vi "1_计算器V1.vi"() -> ()   [LabVIEW 2016]
uses:
  <vilib>/regexp/Match Regular Expression.xnode
panel:
  out "组合框":string(combo)
  in  "按键":T1
  out "Y":string
  out "X":string
  out "B":string
  out "A":string
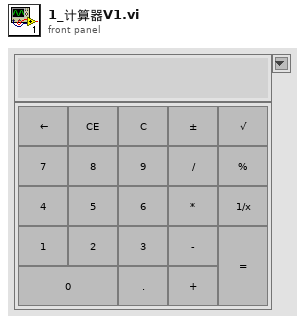
[diagram p1: front panel]
types:
  T1 = cluster{"7":bool, "8":bool, "9":bool, "4":bool, "5":bool, "6":bool, "1":bool, "2":bool, "3":bool, "0":bool, "/":bool, "*":bool, "-":bool, "+":bool, "=":bool, ".":bool, "±":bool, "CE":bool, "C":bool, "←":bool, "√":bool, "1/x":bool, "%":bool}
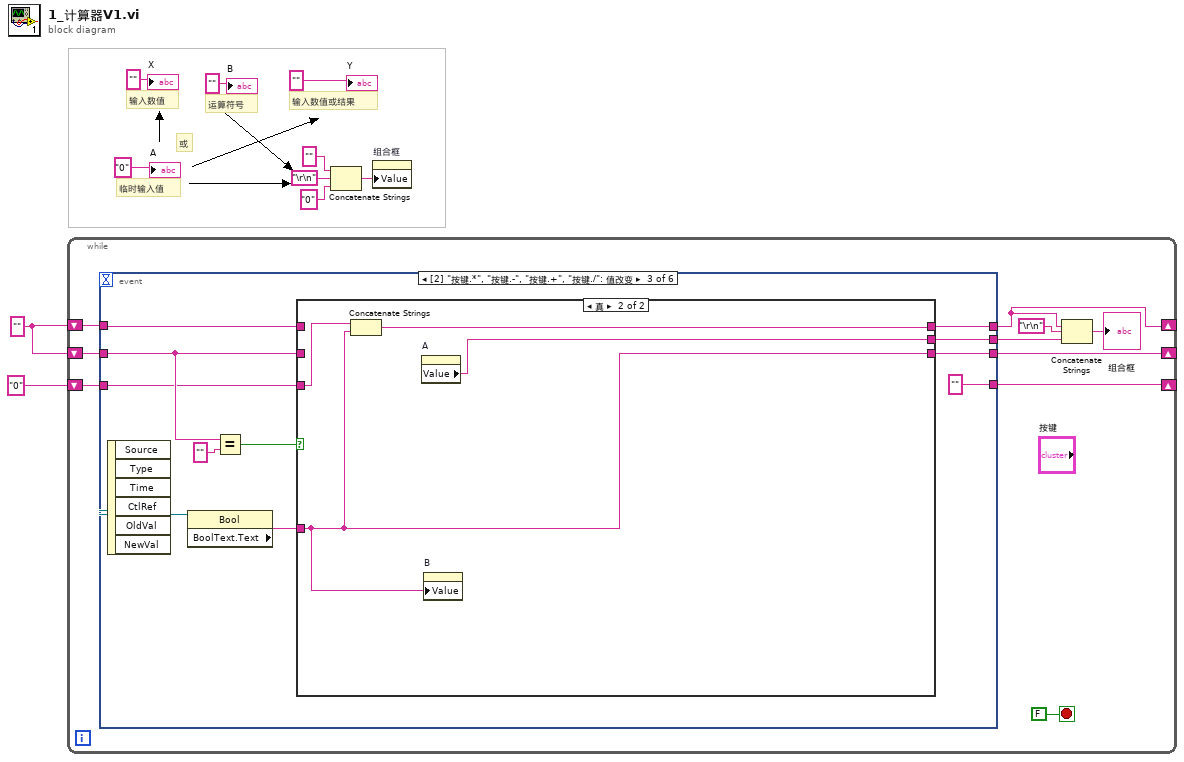
[diagram p0: block diagram]
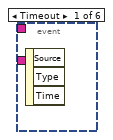
[diagram p2: hidden frame]
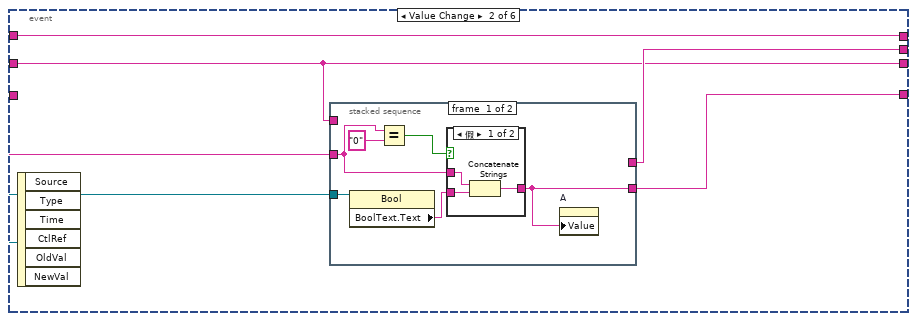
[diagram p3: hidden frame]
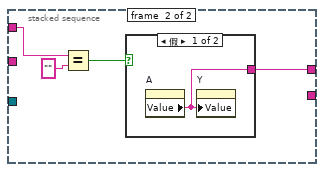
[diagram p5: hidden frame]
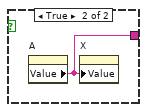
[diagram p6: hidden frame]
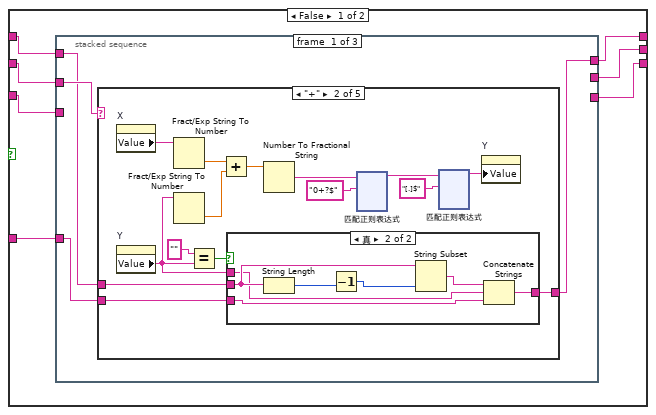
[diagram p7: hidden frame]
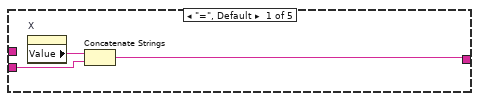
[diagram p8: hidden frame]
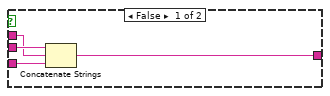
[diagram p9: hidden frame]
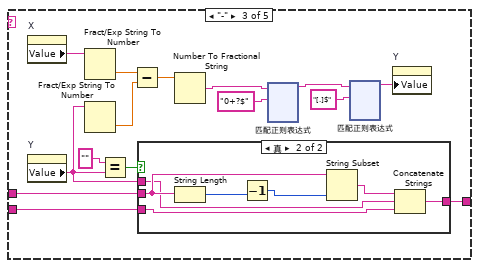
[diagram p10: hidden frame]
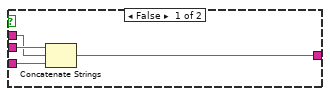
[diagram p11: hidden frame]
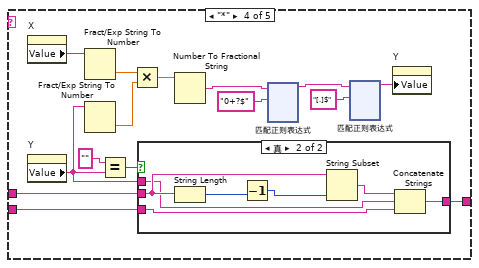
[diagram p12: hidden frame]
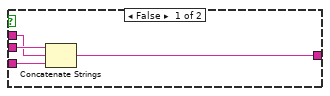
[diagram p13: hidden frame]
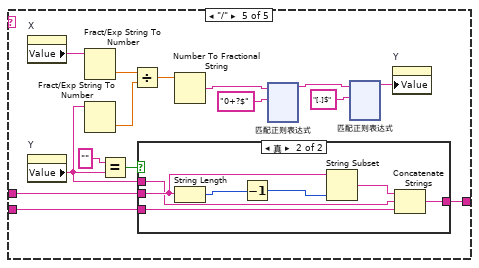
[diagram p14: hidden frame]
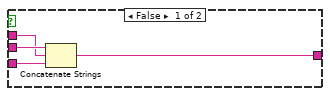
[diagram p15: hidden frame]
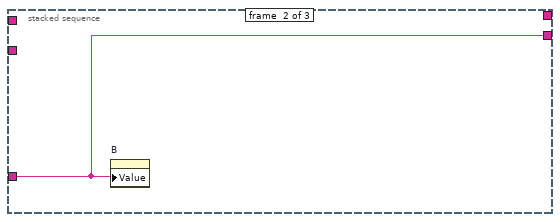
[diagram p16: hidden frame]
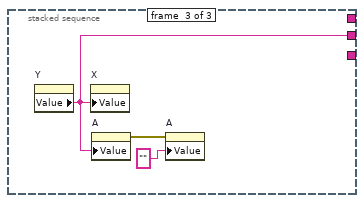
[diagram p17: hidden frame]
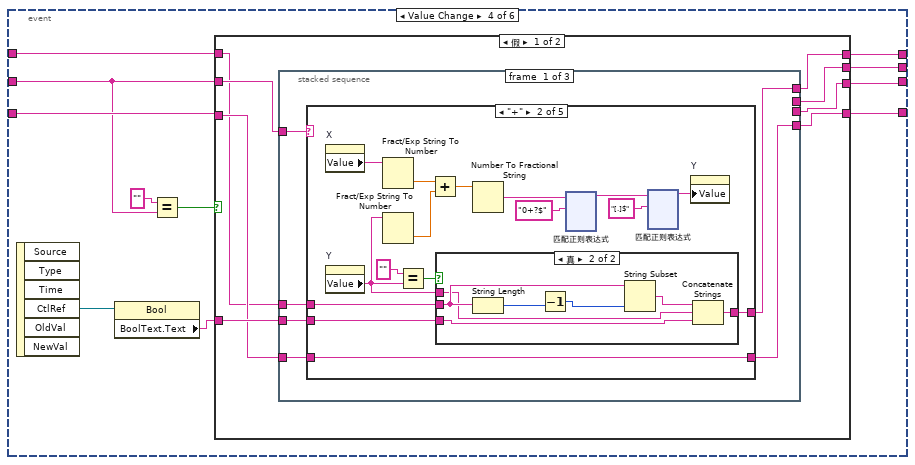
[diagram p18: hidden frame]
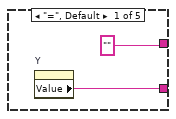
[diagram p19: hidden frame]
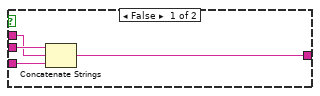
[diagram p20: hidden frame]
diagram:
  w1 = ""
  # "或"
  # "输入数值或结果"
  # "输入数值"
  # "运算符号"
  # "临时输入值"
  n1 = while {
    shift-right: [w18] -> _
    shift-left: "0" -> [w19]
    shift-right: [w16] -> _
    shift-left: w1 -> [w17]
    shift-right: [w12] -> _
    shift-left: w1 -> [w15]
    stop <- FALSE stop-if-true
    n2 = event shown="[2] \"按键.*\", \"按键.-\", \"按键.+\", \"按键./\": 值改变" {
      selector: _ -> [_ _ _ _ _ _]
      dyn-events: _ -> [_ _ _ _ _ _]
      timeout: _ -> [_ _ _ _ _ _]
      tunnel: w19 -> [_ w25 w50 w1098 w2153 w3117]
      tunnel: [_ w24 "" ("BoolText.Text") w1094 w2147 w3112] -> w18
      tunnel: w17 -> [_ w21 w53 w1095 w2149 w3111]
      tunnel: [_ w21 w52 w1092 w2149 w3115] -> w16
      tunnel: w15 -> [_ w23 w43 w1099 w2151 w3114]
      tunnel: [_ w23 w51 w1100 w2151 w3113] -> w12
      tunnel: [_ w22 w44 w1093 w2147 w3116] -> w11
      event Timeout {
        n3 = event-data() -> ()  [unwired: 1 in, 3 out]
      }
      event "按键.7", "按键.8", "按键.9", "按键.4", "按键.5", "按键.6", "按键.1", "按键.2", "按键.3", "按键.0": Value Change {
        n4 = event-data() -> ("CtlRef"=w26:refnum<vi>)  [unwired: 1 in, 5 out]
        n5 = stacked-sequence {
          tunnel: w26 -> [w32 _]
          tunnel: w25 -> [w30 _]
          tunnel: [w27 _] -> w24
          tunnel: w21 -> [_ w40]
          tunnel: [_ w37] -> w22
          frame #0 {
            n6 = property class="Bool"(reference=w32) -> ("BoolText.Text"=w31:string)  [unwired: 1 in, 2 out]
            n7 = Equal?(x=w30, y="0") -> (x = y?=w28:bool)
            n8 = case shown="假" w28 {
              tunnel: w31 -> [w34 w36]
              tunnel: [w33 w36] -> w27
              tunnel: w30 -> [w35 _]
              frame False {
                n9 = Concatenate Strings(w35, w34) -> (w33:string)
              }
              frame True {
              }
            }
            n10 = property on="A" class="Str"("Value"=w27) -> ()  [unwired: 2 in, 2 out]
          }
          frame #1 {
            n11 = Equal?(x=w40, y="") -> (x = y?=w38:bool)
            n12 = case shown="假" w38 {
              tunnel: [w41 w42] -> w37
              frame False {
                n13 = property on="A" class="Str"() -> ("Value"=w41:string)  [unwired: 2 in, 2 out]
                n14 = property on="Y" class="Str"("Value"=w41) -> ()  [unwired: 2 in, 2 out]
              }
              frame True {
                n15 = property on="A" class="Str"() -> ("Value"=w42:string)  [unwired: 2 in, 2 out]
                n16 = property on="X" class="Str"("Value"=w42) -> ()  [unwired: 2 in, 2 out]
              }
            }
          }
        }
      }
      event "按键.*", "按键.-", "按键.+", "按键./": Value Change {
        n17 = event-data() -> ("CtlRef"=w49:refnum<vi>)  [unwired: 1 in, 5 out]
        n18 = property class="Bool"(reference=w49) -> ("BoolText.Text"=w45:string)  [unwired: 1 in, 2 out]
        n19 = Equal?(x=w53, y="") -> (x = y?=w46:bool)
        n20 = case shown="真" w46 {
          tunnel: [w60 w1088] -> w52
          tunnel: w45 -> [w59 w1088]
          tunnel: w43 -> [w58 _]
          tunnel: [w54 w1091] -> w51
          tunnel: w53 -> [w57 _]
          tunnel: w50 -> [w56 w1090]
          tunnel: [w55 w1089] -> w44
          frame False {
            n21 = stacked-sequence {
              tunnel: [_ w1084 _] -> w60
              tunnel: w59 -> [w62 w1084 _]
              tunnel: w58 -> [w61 _ _]
              tunnel: [w63 _ _] -> w54
              tunnel: w57 -> [w64 _ _]
              tunnel: w56 -> [_ _ _]
              tunnel: [_ _ w1085] -> w55
              frame #0 {
                n22 = case shown="\"+\"" w64 {
                  tunnel: w61 -> [_ w77 w329 w584 w838]
                  tunnel: [w65 w76 w328 w583 w837] -> w63
                  tunnel: w62 -> [w66 w75 w330 w582 w836]
                  frame "=", Default {
                    n23 = property on="X" class="Str"() -> ("Value"=w67:string)  [unwired: 2 in, 2 out]
                    n24 = Concatenate Strings(w67, w66) -> (w65:string)
                  }
                  frame "+" {
                    n25 = property on="X" class="Str"() -> ("Value"=w82:string)  [unwired: 2 in, 2 out]
                    n26 = property on="Y" class="Str"() -> ("Value"=w73:string)  [unwired: 2 in, 2 out]
                    n27 = Fract/Exp String To Number(string=w82) -> (number=w81:dbl)  [unwired: 3 in, 1 out]
                    n28 = Fract/Exp String To Number(string=w73) -> (number=w80:dbl)  [unwired: 3 in, 1 out]
                    n29 = Equal?(x="" ("y"), y=w73) -> (x = y?=w78:bool)
                    n30 = Add(x=w81, y=w80) -> (x+y=w79:dbl)
                    n31 = case shown="真" w78 {
                      tunnel: w75 -> [w312 w316]
                      tunnel: w77 -> [w314 w319]
                      tunnel: [w313 w317] -> w76
                      tunnel: w73 -> [w311 w315]
                      frame False {
                        n32 = Concatenate Strings(w314, w311, w312) -> (w313:string)
                      }
                      frame True {
                        n33 = String Length(string=w319) -> (length=w321:i32)
                        n34 = Decrement(x=w321) -> (x-1=w320:i32)
                        n35 = String Subset(string=w319, length (rest)=w320) -> (substring=w318:string)  [unwired: 1 in]
                        n36 = Concatenate Strings(w318, w315, w316) -> (w317:string)
                      }
                    }
                    n37 = Number To Fractional String(number=w79) -> (F-format string=w72:string)  [unwired: 3 in]
                    n38 = xnode "匹配正则表达式"("输入字符串"=w72, "正则表达式"="0+?$") -> ("匹配之前"=w70:string)  [unwired: 4 in, 4 out]
                    n39 = xnode "匹配正则表达式"("输入字符串"=w70, "正则表达式"="[.]$") -> ("匹配之前"=w68:string)  [unwired: 4 in, 4 out]
                    n40 = property on="Y" class="Str"("Value"=w68) -> ()  [unwired: 2 in, 2 out]
                  }
                  frame "-" {
                    n41 = property on="X" class="Str"() -> ("Value"=w331:string)  [unwired: 2 in, 2 out]
                    n42 = property on="Y" class="Str"() -> ("Value"=w327:string)  [unwired: 2 in, 2 out]
                    n43 = Fract/Exp String To Number(string=w331) -> (number=w332:dbl)  [unwired: 3 in, 1 out]
                    n44 = Fract/Exp String To Number(string=w327) -> (number=w333:dbl)  [unwired: 3 in, 1 out]
                    n45 = Equal?(x="" ("y"), y=w327) -> (x = y?=w335:bool)
                    n46 = Subtract(x=w332, y=w333) -> (x-y=w334:dbl)
                    n47 = case shown="真" w335 {
                      tunnel: w330 -> [w566 w570]
                      tunnel: w329 -> [w568 w573]
                      tunnel: [w567 w572] -> w328
                      tunnel: w327 -> [w565 w569]
                      frame False {
                        n48 = Concatenate Strings(w568, w565, w566) -> (w567:string)
                      }
                      frame True {
                        n49 = String Length(string=w573) -> (length=w575:i32)
                        n50 = Decrement(x=w575) -> (x-1=w574:i32)
                        n51 = String Subset(string=w573, length (rest)=w574) -> (substring=w571:string)  [unwired: 1 in]
                        n52 = Concatenate Strings(w571, w569, w570) -> (w572:string)
                      }
                    }
                    n53 = Number To Fractional String(number=w334) -> (F-format string=w323:string)  [unwired: 3 in]
                    n54 = xnode "匹配正则表达式"("输入字符串"=w323, "正则表达式"="0+?$") -> ("匹配之前"=w325:string)  [unwired: 4 in, 4 out]
                    n55 = xnode "匹配正则表达式"("输入字符串"=w325, "正则表达式"="[.]$") -> ("匹配之前"=w322:string)  [unwired: 4 in, 4 out]
                    n56 = property on="Y" class="Str"("Value"=w322) -> ()  [unwired: 2 in, 2 out]
                  }
                  frame "*" {
                    n57 = property on="X" class="Str"() -> ("Value"=w585:string)  [unwired: 2 in, 2 out]
                    n58 = property on="Y" class="Str"() -> ("Value"=w581:string)  [unwired: 2 in, 2 out]
                    n59 = Fract/Exp String To Number(string=w585) -> (number=w586:dbl)  [unwired: 3 in, 1 out]
                    n60 = Fract/Exp String To Number(string=w581) -> (number=w587:dbl)  [unwired: 3 in, 1 out]
                    n61 = Equal?(x="" ("y"), y=w581) -> (x = y?=w589:bool)
                    n62 = Multiply(x=w586, y=w587) -> (x*y=w588:dbl)
                    n63 = case shown="真" w589 {
                      tunnel: w582 -> [w820 w824]
                      tunnel: w584 -> [w822 w827]
                      tunnel: [w821 w826] -> w583
                      tunnel: w581 -> [w819 w823]
                      frame False {
                        n64 = Concatenate Strings(w822, w819, w820) -> (w821:string)
                      }
                      frame True {
                        n65 = String Length(string=w827) -> (length=w829:i32)
                        n66 = Decrement(x=w829) -> (x-1=w828:i32)
                        n67 = String Subset(string=w827, length (rest)=w828) -> (substring=w825:string)  [unwired: 1 in]
                        n68 = Concatenate Strings(w825, w823, w824) -> (w826:string)
                      }
                    }
                    n69 = Number To Fractional String(number=w588) -> (F-format string=w577:string)  [unwired: 3 in]
                    n70 = xnode "匹配正则表达式"("输入字符串"=w577, "正则表达式"="0+?$") -> ("匹配之前"=w579:string)  [unwired: 4 in, 4 out]
                    n71 = xnode "匹配正则表达式"("输入字符串"=w579, "正则表达式"="[.]$") -> ("匹配之前"=w576:string)  [unwired: 4 in, 4 out]
                    n72 = property on="Y" class="Str"("Value"=w576) -> ()  [unwired: 2 in, 2 out]
                  }
                  frame "/" {
                    n73 = property on="X" class="Str"() -> ("Value"=w839:string)  [unwired: 2 in, 2 out]
                    n74 = property on="Y" class="Str"() -> ("Value"=w835:string)  [unwired: 2 in, 2 out]
                    n75 = Fract/Exp String To Number(string=w839) -> (number=w840:dbl)  [unwired: 3 in, 1 out]
                    n76 = Fract/Exp String To Number(string=w835) -> (number=w841:dbl)  [unwired: 3 in, 1 out]
                    n77 = Equal?(x="" ("y"), y=w835) -> (x = y?=w843:bool)
                    n78 = Divide(x=w840, y=w841) -> (x/y=w842:dbl)
                    n79 = case shown="真" w843 {
                      tunnel: w836 -> [w1074 w1078]
                      tunnel: w838 -> [w1076 w1081]
                      tunnel: [w1075 w1080] -> w837
                      tunnel: w835 -> [w1073 w1077]
                      frame False {
                        n80 = Concatenate Strings(w1076, w1073, w1074) -> (w1075:string)
                      }
                      frame True {
                        n81 = String Length(string=w1081) -> (length=w1083:i32)
                        n82 = Decrement(x=w1083) -> (x-1=w1082:i32)
                        n83 = String Subset ("截取字符串")(string=w1081, length (rest)=w1082) -> (substring=w1079:string)  [unwired: 1 in]
                        n84 = Concatenate Strings(w1079, w1077, w1078) -> (w1080:string)
                      }
                    }
                    n85 = Number To Fractional String(number=w842) -> (F-format string=w831:string)  [unwired: 3 in]
                    n86 = xnode "匹配正则表达式"("输入字符串"=w831, "正则表达式"="0+?$") -> ("匹配之前"=w833:string)  [unwired: 4 in, 4 out]
                    n87 = xnode "匹配正则表达式"("输入字符串"=w833, "正则表达式"="[.]$") -> ("匹配之前"=w830:string)  [unwired: 4 in, 4 out]
                    n88 = property on="Y" class="Str"("Value"=w830) -> ()  [unwired: 2 in, 2 out]
                  }
                }
              }
              frame #1 {
                n89 = property on="B" class="Str"("Value"=w1084) -> ()  [unwired: 2 in, 2 out]
              }
              frame #2 {
                n90 = property on="Y" class="Str"() -> ("Value"=w1085:string)  [unwired: 2 in, 2 out]
                n91 = property on="X" class="Str"("Value"=w1085) -> ()  [unwired: 2 in, 2 out]
                n92 = property on="A" class="Str"("Value"=w1085) -> (error out=w1086:errorcluster)  [unwired: 2 in, 1 out]
                n93 = property on="A" class="Str"(error in=w1086, "Value"="" ("C")) -> ()  [unwired: 1 in, 2 out]
              }
            }
          }
          frame True {
            n94 = Concatenate Strings(w1090, w1088) -> (w1091:string)
            n95 = property on="A" class="Str"() -> ("Value"=w1089:string)  [unwired: 2 in, 2 out]
            n96 = property on="B" class="Str"("Value"=w1088) -> ()  [unwired: 2 in, 2 out]
          }
        }
      }
      event "按键.=": Value Change {
        n97 = event-data() -> ("CtlRef"=w1097:refnum<vi>)  [unwired: 1 in, 5 out]
        n98 = property class="Bool"(reference=w1097) -> ("BoolText.Text"=w1096:string)  [unwired: 1 in, 2 out]
        n99 = Equal?(x="", y=w1095) -> (x = y?=w1101:bool)
        n100 = case shown="假" w1101 {
          tunnel: [w1108 ""] -> w1100
          tunnel: w1099 -> [w1103 _]
          tunnel: w1098 -> [w1104 w2143]
          tunnel: [w1107 w2144] -> w1092
          tunnel: w1096 -> [w1109 w2144]
          tunnel: w1095 -> [w1110 _]
          tunnel: [w1106 w2143] -> w1094
          tunnel: [w1105 w2143] -> w1093
          frame False {
            n101 = stacked-sequence {
              tunnel: w1110 -> [w1116 _ _]
              tunnel: w1109 -> [w1115 w2139 _]
              tunnel: w1103 -> [w1114 _ _]
              tunnel: [w1113 _ _] -> w1108
              tunnel: [_ w2139 _] -> w1107
              tunnel: w1104 -> [w1112 _ _]
              tunnel: [w1111 _ _] -> w1106
              tunnel: [_ _ w2141] -> w1105
              frame #0 {
                n102 = case shown="\"+\"" w1116 {
                  tunnel: w1114 -> [_ w1129 w1382 w1638 w1893]
                  tunnel: ["" w1128 w1381 w1637 w1892] -> w1113
                  tunnel: w1115 -> [_ w1127 w1383 w1636 w1891]
                  tunnel: w1112 -> [_ w1124 w1379 w1634 w1884]
                  tunnel: [w1117 w1124 w1379 w1634 w1884] -> w1111
                  frame "=", Default {
                    n103 = property on="Y" class="Str"() -> ("Value"=w1117:string)  [unwired: 2 in, 2 out]
                  }
                  frame "+" {
                    n104 = property on="X" class="Str"() -> ("Value"=w1134:string)  [unwired: 2 in, 2 out]
                    n105 = property on="Y" class="Str"() -> ("Value"=w1125:string)  [unwired: 2 in, 2 out]
                    n106 = Fract/Exp String To Number(string=w1134) -> (number=w1133:dbl)  [unwired: 3 in, 1 out]
                    n107 = Fract/Exp String To Number(string=w1125) -> (number=w1132:dbl)  [unwired: 3 in, 1 out]
                    n108 = Equal?(x="" ("y"), y=w1125) -> (x = y?=w1130:bool)
                    n109 = Add(x=w1133, y=w1132) -> (x+y=w1131:dbl)
                    n110 = case shown="真" w1130 {
                      tunnel: w1127 -> [w1364 w1368]
                      tunnel: w1129 -> [w1366 w1371]
                      tunnel: [w1365 w1369] -> w1128
                      tunnel: w1125 -> [w1363 w1367]
                      frame False {
                        n111 = Concatenate Strings(w1366, w1363, w1364) -> (w1365:string)
                      }
                      frame True {
                        n112 = String Length(string=w1371) -> (length=w1373:i32)
                        n113 = Decrement(x=w1373) -> (x-1=w1372:i32)
                        n114 = String Subset(string=w1371, length (rest)=w1372) -> (substring=w1370:string)  [unwired: 1 in]
                        n115 = Concatenate Strings(w1370, w1367, w1368) -> (w1369:string)
                      }
                    }
                    n116 = Number To Fractional String(number=w1131) -> (F-format string=w1120:string)  [unwired: 3 in]
                    n117 = xnode "匹配正则表达式"("输入字符串"=w1120, "正则表达式"="0+?$") -> ("匹配之前"=w1122:string)  [unwired: 4 in, 4 out]
                    n118 = xnode "匹配正则表达式"("输入字符串"=w1122, "正则表达式"="[.]$") -> ("匹配之前"=w1119:string)  [unwired: 4 in, 4 out]
                    n119 = property on="Y" class="Str"("Value"=w1119) -> ()  [unwired: 2 in, 2 out]
                  }
                  frame "-" {
                    n120 = property on="X" class="Str"() -> ("Value"=w1384:string)  [unwired: 2 in, 2 out]
                    n121 = property on="Y" class="Str"() -> ("Value"=w1380:string)  [unwired: 2 in, 2 out]
                    n122 = Fract/Exp String To Number(string=w1384) -> (number=w1385:dbl)  [unwired: 3 in, 1 out]
                    n123 = Fract/Exp String To Number(string=w1380) -> (number=w1386:dbl)  [unwired: 3 in, 1 out]
                    n124 = Equal?(x="" ("y"), y=w1380) -> (x = y?=w1388:bool)
                    n125 = Subtract(x=w1385, y=w1386) -> (x-y=w1387:dbl)
                    n126 = case shown="真" w1388 {
                      tunnel: w1383 -> [w1619 w1623]
                      tunnel: w1382 -> [w1621 w1626]
                      tunnel: [w1620 w1625] -> w1381
                      tunnel: w1380 -> [w1618 w1622]
                      frame False {
                        n127 = Concatenate Strings(w1621, w1618, w1619) -> (w1620:string)
                      }
                      frame True {
                        n128 = String Length(string=w1626) -> (length=w1628:i32)
                        n129 = Decrement(x=w1628) -> (x-1=w1627:i32)
                        n130 = String Subset(string=w1626, length (rest)=w1627) -> (substring=w1624:string)  [unwired: 1 in]
                        n131 = Concatenate Strings(w1624, w1622, w1623) -> (w1625:string)
                      }
                    }
                    n132 = Number To Fractional String(number=w1387) -> (F-format string=w1375:string)  [unwired: 3 in]
                    n133 = xnode "匹配正则表达式"("输入字符串"=w1375, "正则表达式"="0+?$") -> ("匹配之前"=w1377:string)  [unwired: 4 in, 4 out]
                    n134 = xnode "匹配正则表达式"("输入字符串"=w1377, "正则表达式"="[.]$") -> ("匹配之前"=w1374:string)  [unwired: 4 in, 4 out]
                    n135 = property on="Y" class="Str"("Value"=w1374) -> ()  [unwired: 2 in, 2 out]
                  }
                  frame "*" {
                    n136 = property on="X" class="Str"() -> ("Value"=w1639:string)  [unwired: 2 in, 2 out]
                    n137 = property on="Y" class="Str"() -> ("Value"=w1635:string)  [unwired: 2 in, 2 out]
                    n138 = Fract/Exp String To Number(string=w1639) -> (number=w1640:dbl)  [unwired: 3 in, 1 out]
                    n139 = Fract/Exp String To Number(string=w1635) -> (number=w1641:dbl)  [unwired: 3 in, 1 out]
                    n140 = Equal?(x="" ("y"), y=w1635) -> (x = y?=w1643:bool)
                    n141 = Multiply(x=w1640, y=w1641) -> (x*y=w1642:dbl)
                    n142 = case shown="真" w1643 {
                      tunnel: w1636 -> [w1874 w1878]
                      tunnel: w1638 -> [w1876 w1881]
                      tunnel: [w1875 w1880] -> w1637
                      tunnel: w1635 -> [w1873 w1877]
                      frame False {
                        n143 = Concatenate Strings(w1876, w1873, w1874) -> (w1875:string)
                      }
                      frame True {
                        n144 = String Length(string=w1881) -> (length=w1883:i32)
                        n145 = Decrement(x=w1883) -> (x-1=w1882:i32)
                        n146 = String Subset(string=w1881, length (rest)=w1882) -> (substring=w1879:string)  [unwired: 1 in]
                        n147 = Concatenate Strings(w1879, w1877, w1878) -> (w1880:string)
                      }
                    }
                    n148 = Number To Fractional String(number=w1642) -> (F-format string=w1630:string)  [unwired: 3 in]
                    n149 = xnode "匹配正则表达式"("输入字符串"=w1630, "正则表达式"="0+?$") -> ("匹配之前"=w1632:string)  [unwired: 4 in, 4 out]
                    n150 = xnode "匹配正则表达式"("输入字符串"=w1632, "正则表达式"="[.]$") -> ("匹配之前"=w1629:string)  [unwired: 4 in, 4 out]
                    n151 = property on="Y" class="Str"("Value"=w1629) -> ()  [unwired: 2 in, 2 out]
                  }
                  frame "/" {
                    n152 = property on="X" class="Str"() -> ("Value"=w1894:string)  [unwired: 2 in, 2 out]
                    n153 = property on="Y" class="Str"() -> ("Value"=w1890:string)  [unwired: 2 in, 2 out]
                    n154 = Fract/Exp String To Number(string=w1894) -> (number=w1895:dbl)  [unwired: 3 in, 1 out]
                    n155 = Fract/Exp String To Number(string=w1890) -> (number=w1896:dbl)  [unwired: 3 in, 1 out]
                    n156 = Equal?(x="" ("y"), y=w1890) -> (x = y?=w1898:bool)
                    n157 = Divide(x=w1895, y=w1896) -> (x/y=w1897:dbl)
                    n158 = case shown="真" w1898 {
                      tunnel: w1891 -> [w2129 w2133]
                      tunnel: w1893 -> [w2131 w2136]
                      tunnel: [w2130 w2135] -> w1892
                      tunnel: w1890 -> [w2128 w2132]
                      frame False {
                        n159 = Concatenate Strings(w2131, w2128, w2129) -> (w2130:string)
                      }
                      frame True {
                        n160 = String Length(string=w2136) -> (length=w2138:i32)
                        n161 = Decrement(x=w2138) -> (x-1=w2137:i32)
                        n162 = String Subset(string=w2136, length (rest)=w2137) -> (substring=w2134:string)  [unwired: 1 in]
                        n163 = Concatenate Strings(w2134, w2132, w2133) -> (w2135:string)
                      }
                    }
                    n164 = Number To Fractional String(number=w1897) -> (F-format string=w1886:string)  [unwired: 3 in]
                    n165 = xnode "匹配正则表达式"("输入字符串"=w1886, "正则表达式"="0+?$") -> ("匹配之前"=w1888:string)  [unwired: 4 in, 4 out]
                    n166 = xnode "匹配正则表达式"("输入字符串"=w1888, "正则表达式"="[.]$") -> ("匹配之前"=w1885:string)  [unwired: 4 in, 4 out]
                    n167 = property on="Y" class="Str"("Value"=w1885) -> ()  [unwired: 2 in, 2 out]
                  }
                }
              }
              frame #1 {
                n168 = property on="B" class="Str"("Value"=w2139) -> ()  [unwired: 2 in, 2 out]
              }
              frame #2 {
                n169 = property on="Y" class="Str"() -> ("Value"=w2141:string)  [unwired: 2 in, 2 out]
                n170 = property on="X" class="Str"("Value"=w2141) -> ()  [unwired: 2 in, 2 out]
                n171 = property on="A" class="Str"("Value"=w2141) -> (error out=w2140:errorcluster)  [unwired: 2 in, 1 out]
                n172 = property on="A" class="Str"(error in=w2140, "Value"="" ("C")) -> ()  [unwired: 1 in, 2 out]
              }
            }
          }
          frame True {
            n173 = property on="A" class="Str"("Value"=w2143) -> ()  [unwired: 2 in, 2 out]
          }
        }
      }
      event "按键..", "按键.±", "按键.√", "按键.1/x", "按键.%": Value Change {
        n174 = event-data() -> ("CtlRef"=w2152:refnum<vi>)  [unwired: 1 in, 5 out]
        n175 = property class="Bool"(reference=w2152) -> ("BoolText.Text"=w2146:string)  [unwired: 1 in, 2 out]
        n176 = case shown="\"%\"" w2146 {
          tunnel: w2153 -> [w2163 w2396 w2628 w2867 w2882]
          tunnel: w2146 -> [_ _ _ w2866 _]
          tunnel: [w2156 w2392 w2631 w2865 w2875] -> w2147
          frame "±", Default {
            n177 = Fract/Exp String To Number(string=w2163) -> (number=w2162:dbl)  [unwired: 3 in, 1 out]
            n178 = Negate(x=w2162) -> (-x=w2161:dbl)
            n179 = Number To Fractional String(number=w2161) -> (F-format string=w2157:string)  [unwired: 3 in]
            n180 = xnode "匹配正则表达式"("输入字符串"=w2157, "正则表达式"="0+?$") -> ("匹配之前"=w2159:string)  [unwired: 4 in, 4 out]
            n181 = xnode "匹配正则表达式"("输入字符串"=w2159, "正则表达式"="[.]$") -> ("匹配之前"=w2156:string)  [unwired: 4 in, 4 out]
          }
          frame "1/x" {
            n182 = Fract/Exp String To Number(string=w2396) -> (number=w2395:dbl)  [unwired: 3 in, 1 out]
            n183 = Reciprocal(x=w2395) -> (1/x=w2394:dbl)
            n184 = Number To Fractional String(number=w2394) -> (F-format string=w2393:string)  [unwired: 3 in]
            n185 = xnode "匹配正则表达式"("输入字符串"=w2393, "正则表达式"="0+?$") -> ("匹配之前"=w2398:string)  [unwired: 4 in, 4 out]
            n186 = xnode "匹配正则表达式"("输入字符串"=w2398, "正则表达式"="[.]$") -> ("匹配之前"=w2392:string)  [unwired: 4 in, 4 out]
          }
          frame "%" {
            n187 = Fract/Exp String To Number(string=w2628) -> (number=w2630:dbl)  [unwired: 3 in, 1 out]
            n188 = Divide(x=w2630, y=100.0) -> (x/y=w2633:dbl)
            n189 = Number To Fractional String(number=w2633) -> (F-format string=w2632:string)  [unwired: 3 in]
            n190 = xnode "匹配正则表达式"("输入字符串"=w2632, "正则表达式"="0+?$") -> ("匹配之前"=w2635:string)  [unwired: 4 in, 4 out]
            n191 = xnode "匹配正则表达式"("输入字符串"=w2635, "正则表达式"="[.]$") -> ("匹配之前"=w2631:string)  [unwired: 4 in, 4 out]
          }
          frame "." {
            n192 = Search and Replace String(input string=w2867, search string="." ("搜索字符串")) -> (number of replacements=w2869:i32)  [unwired: 6 in, 3 out]
            n193 = Equal To 0?(x=w2869) -> (x = 0?=w2868:bool)
            n194 = case shown="真" w2868 {
              tunnel: w2867 -> [w2871 w2874]
              tunnel: w2866 -> [_ w2872]
              tunnel: [w2871 w2873] -> w2865
              frame False {
              }
              frame True {
                n195 = Concatenate Strings(w2874, w2872) -> (w2873:string)
              }
            }
          }
          frame "√" {
            n196 = Fract/Exp String To Number(string=w2882) -> (number=w2881:dbl)  [unwired: 3 in, 1 out]
            n197 = Square Root(x=w2881) -> (sqrt(x)=w2877:dbl)
            n198 = Number To Fractional String(number=w2877) -> (F-format string=w2876:string)  [unwired: 3 in]
            n199 = xnode "匹配正则表达式"("输入字符串"=w2876, "正则表达式"="0+?$") -> ("匹配之前"=w2879:string)  [unwired: 4 in, 4 out]
            n200 = xnode "匹配正则表达式"("输入字符串"=w2879, "正则表达式"="[.]$") -> ("匹配之前"=w2875:string)  [unwired: 4 in, 4 out]
          }
        }
        n201 = Equal?(x=w2149, y="") -> (x = y?=w2148:bool)
        n202 = property on="A" class="Str"("Value"=w2147) -> ()  [unwired: 2 in, 2 out]
        n203 = case shown="真" w2148 {
          tunnel: w2147 -> [w2154 w2155]
          frame False {
            n204 = property on="Y" class="Str"("Value"=w2154) -> ()  [unwired: 2 in, 2 out]
          }
          frame True {
            n205 = property on="X" class="Str"("Value"=w2155) -> ()  [unwired: 2 in, 2 out]
          }
        }
      }
      event "按键.C", "按键.←", "按键.CE": Value Change {
        n206 = event-data() -> ("CtlRef"=w3119:refnum<vi>)  [unwired: 1 in, 5 out]
        n207 = property class="Bool"(reference=w3119) -> ("BoolText.Text"=w3118:string)  [unwired: 1 in, 2 out]
        n208 = case shown="\"C\"" w3118 {
          tunnel: w3117 -> [w3120 w3134 w3142]
          tunnel: w3111 -> [w3123 w3133 w3140]
          tunnel: [w3126 w3132 w3141] -> w3112
          tunnel: ["" w3132 w3141] -> w3116
          tunnel: ["" w3133 w3140] -> w3115
          tunnel: w3114 -> [_ w3131 w3139]
          tunnel: ["" w3131 w3139] -> w3113
          frame "C" {
            w3121 = "" ("甲")
            n209 = Equal?(x=w3123, y="") -> (x = y?=w3127:bool)
            n210 = case shown="假" w3127 {
              tunnel: [w3129 w3130] -> w3126
              tunnel: w3120 -> [_ _]
              frame False {
                w3129 = ""
                n211 = property on="Y" class="Str"("Value"=w3129) -> ()  [unwired: 2 in, 2 out]
                n212 = property on="A" class="Str"("Value"=w3129) -> ()  [unwired: 2 in, 2 out]
              }
              frame True {
                w3130 = ""
                n213 = property on="X" class="Str"("Value"=w3130) -> ()  [unwired: 2 in, 2 out]
                n214 = property on="A" class="Str"("Value"=w3130) -> ()  [unwired: 2 in, 2 out]
              }
            }
            n215 = property on="Y" class="Str"("Value"=w3121) -> ()  [unwired: 2 in, 2 out]
            n216 = property on="X" class="Str"("Value"=w3121) -> ()  [unwired: 2 in, 2 out]
          }
          frame "CE" {
            n217 = Equal?(x=w3133, y="") -> (x = y?=w3135:bool)
            n218 = case shown="真" w3135 {
              tunnel: [w3137 w3138] -> w3132
              tunnel: w3134 -> [_ _]
              frame False {
                w3137 = ""
                n219 = property on="Y" class="Str"("Value"=w3137) -> ()  [unwired: 2 in, 2 out]
                n220 = property on="A" class="Str"("Value"=w3137) -> ()  [unwired: 2 in, 2 out]
              }
              frame True {
                w3138 = ""
                n221 = property on="X" class="Str"("Value"=w3138) -> ()  [unwired: 2 in, 2 out]
                n222 = property on="A" class="Str"("Value"=w3138) -> ()  [unwired: 2 in, 2 out]
              }
            }
          }
          frame "←", Default {
            n223 = Equal?(x=w3140, y="") -> (x = y?=w3144:bool)
            n224 = case shown="假" w3144 {
              tunnel: [w3146 w3150] -> w3141
              tunnel: w3142 -> [w3145 w3149]
              frame False {
                n225 = String Length(string=w3145) -> (length=w3148:i32)
                n226 = Decrement(x=w3148) -> (x-1=w3147:i32)
                n227 = String Subset(string=w3145, length (rest)=w3147) -> (substring=w3146:string)  [unwired: 1 in]
                n228 = property on="A" class="Str"("Value"=w3146) -> ()  [unwired: 2 in, 2 out]
                n229 = property on="Y" class="Str"("Value"=w3146) -> ()  [unwired: 2 in, 2 out]
              }
              frame True {
                n230 = String Length(string=w3149) -> (length=w3152:i32)
                n231 = Decrement(x=w3152) -> (x-1=w3151:i32)
                n232 = String Subset(string=w3149, length (rest)=w3151) -> (substring=w3150:string)  [unwired: 1 in]
                n233 = property on="X" class="Str"("Value"=w3150) -> ()  [unwired: 2 in, 2 out]
                n234 = property on="A" class="Str"("Value"=w3150) -> ()  [unwired: 2 in, 2 out]
              }
            }
          }
        }
      }
    }
    n235 = Concatenate Strings(w12, "\r\n", w11) -> (→"组合框":string)
  }
  n236 = Concatenate Strings("" ("字符串"), "\r\n", "0" ("字符串")) -> (w5:string)
  n237 = property on="组合框" class="CmbBox"("Value"=w5) -> ()  [unwired: 2 in, 2 out]
  "A" <- "0" ("C")
  "B" <- "" ("D")
  "X" <- "" ("甲")
  "Y" <- "" ("甲")
